vi "FPGA_AIERRInvalidAnalogChannel.vi"(8 "error in (no error)":errorcluster, 9 "Additional Depth":i32) -> (0 "error out":errorcluster)   [LabVIEW 2017]
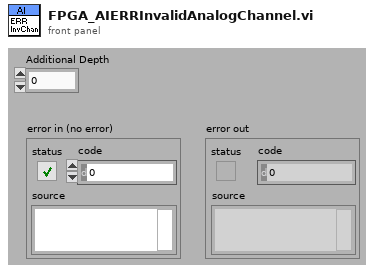
[diagram p1: front panel]
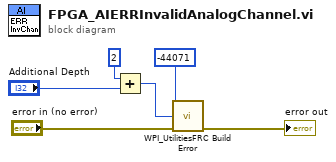
[diagram p0: block diagram]
diagram:
  n1 = Add(x=2 ("chain levels to remove (1)"), y="Additional Depth") -> (x+y=w3:i32)
  n2 = call <vilib>:"WPI_UtilitiesFRC Build Error.vi"("error code"=-44071 ("code"), "chain levels to remove (1)"=w3, "error in (no error)"="error in (no error)") -> ("error out"=→"error out":errorcluster)  [unwired: 2 in, 10 out]
